vi "Event Handler.vi"(8 "error in (no error)":errorcluster, 10 "Stop Event Handler":refnum<user-event>, 11 "SwipeMenu in":refnum<class "SwipeMenu.lvclass">) -> (0 "error out":errorcluster)   [LabVIEW 2020, in "SwipeMenu.lvclass"]
doc: "The <b>Event Handler VI</b> is a dynamic dispatch VI that should be overwritten if events are needed to create the enhanced QControl. \n\nBy inheriting from the main Control.lvclass the overwritten <b>Event Handler VI</b> will be launched asynchronously in the initialization of the QControl.\n<b> </b> <b> </b>\n©2016 Q Software Innovations, LLC (QSI)\nwritten by Quentin Alldredge\nproduced in LabVIEW 2015\n\nsupport@qsoftwareinnovations.com\nwww.qsoftwareinnovations.com\n\nAll rights reserved.\n\nRedistribution and use in source and binary forms, with or without modification, are permitted provided that the following conditions are met:\n\n * Redistributions of source code must retain the above copyright notice, this list of conditions and the following disclaimer.\n * Redistributions in binary form must reproduce the above copyright notice, this list of conditions and the following disclaimer in the documentation and/or other materials provided with the distribution.\n * Neither the name of Q Software Innovations, LLC. nor the names of its contributors may be used to endorse or promote products derived from this software without specific prior written permission.\n\nTHIS SOFTWARE IS PROVIDED BY THE COPYRIGHT HOLDERS AND CONTRIBUTORS \"AS IS\" AND ANY EXPRESS OR IMPLIED WARRANTIES, INCLUDING, BUT NOT LIMITED TO, THE IMPLIED WARRANTIES OF MERCHANTABILITY AND FITNESS FOR A PARTICULAR PURPOSE ARE DISCLAIMED. IN NO EVENT SHALL THE COPYRIGHT OWNER OR CONTRIBUTORS BE LIABLE FOR ANY DIRECT, INDIRECT, INCIDENTAL, SPECIAL, EXEMPLARY, OR CONSEQUENTIAL DAMAGES (INCLUDING, BUT NOT LIMITED TO, PROCUREMENT OF SUBSTITUTE GOODS OR SERVICES; LOSS OF USE, DATA, OR PROFITS; OR BUSINESS INTERRUPTION) HOWEVER CAUSED AND ON ANY THEORY OF LIABILITY, WHETHER IN CONTRACT, STRICT LIABILITY, OR TORT (INCLUDING NEGLIGENCE OR OTHERWISE) ARISING IN ANY WAY OUT OF THE USE OF THIS SOFTWARE, EVEN IF ADVISED OF THE POSSIBILITY OF SUCH DAMAGE."
uses:
  SwipeMenu.lvclass
  Menu Cluster.ctl
  Demo Buttons/Test Button.ctl
  Demo Buttons/About Button.ctl
  Demo Buttons/Dismiss Popup.ctl
  Demo Buttons/QSI Button.ctl
  Demo Buttons/Checkbox Demo Button.ctl
  Demo Buttons/Dialogs Demo Button.ctl
  Demo Buttons/Example SubMenu Button.ctl
  Demo Buttons/Filter Clicks.ctl
  Demo Buttons/Listbox Demo Button.ctl
  Demo Buttons/OSK Demo Button.ctl
  Demo Buttons/Scrollbar Demo Button.ctl
  Demo Buttons/String Scrollbar Demo Button.ctl
  Demo Buttons/Swipe Scroll Button.ctl
  Demo Buttons/Swipe Select Button.ctl
  Left.ctl
  Right.ctl
  <vilib>/Utility/miscctls.llb/LVPointTypeDef.ctl
  SwipeMenu.lvclass/SwipeMenu.ctl
panel:
  in  "Left":T1
  in  "Menu Cluster":T2
  in  "Right":T17
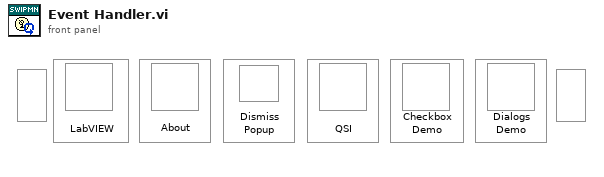
[diagram p1: front panel]
types:
  T1 = typedef "SwipeMenu.lvclass/Left.ctl" = bool
  T2 = typedef "SwipeMenu.lvclass/Menu Cluster.ctl" = cluster{"LabVIEW":T3, "About":T4, "Dismiss Popup":T5, "QSI":T6, "Checkboxes Demo":T7, "Dialog Demo":T8, "Submenu Demo":T9, "Filter Clicks":T10, "Listboxes Demo":T11, "OSK Demo":T12, "Scrollbar Demo":T13, "String Demo":T14, "Swipe Scroll":T15, "Swipe Select":T16, "LabVIEW 2":T3, "About 2":T4, "Dismiss Popup 2":T5, "QSI 2":T6, "Checkboxes Demo 2":T7, "Dialog Demo 2":T8, "Submenu Demo 2":T9, "Filter Clicks 2":T10, "Listboxes Demo 2":T11, "OSK Demo 2":T12, "Scrollbar Demo 2":T13, "String Demo 2":T14, "Swipe Scroll 2":T15, "Swipe Select 2":T16}
  T3 = typedef "Test Button.ctl" = bool
  T4 = typedef "About Button.ctl" = bool
  T5 = typedef "Dismiss Popup.ctl" = bool
  T6 = typedef "QSI Button.ctl" = bool
  T7 = typedef "Checkbox Demo Button.ctl" = bool
  T8 = typedef "Dialogs Demo Button.ctl" = bool
  T9 = typedef "Example SubMenu Button.ctl" = bool
  T10 = typedef "Filter Clicks.ctl" = bool
  T11 = typedef "Listbox Demo Button.ctl" = bool
  T12 = typedef "OSK Demo Button.ctl" = bool
  T13 = typedef "Scrollbar Demo Button.ctl" = bool
  T14 = typedef "String Scrollbar Demo Button.ctl" = bool
  T15 = typedef "Swipe Scroll Button.ctl" = bool
  T16 = typedef "Swipe Select Button.ctl" = bool
  T17 = typedef "SwipeMenu.lvclass/Right.ctl" = bool
  T18 = typedef "LVPointTypeDef.ctl" = cluster{"Horizontal":i16, "Vertical":i16}
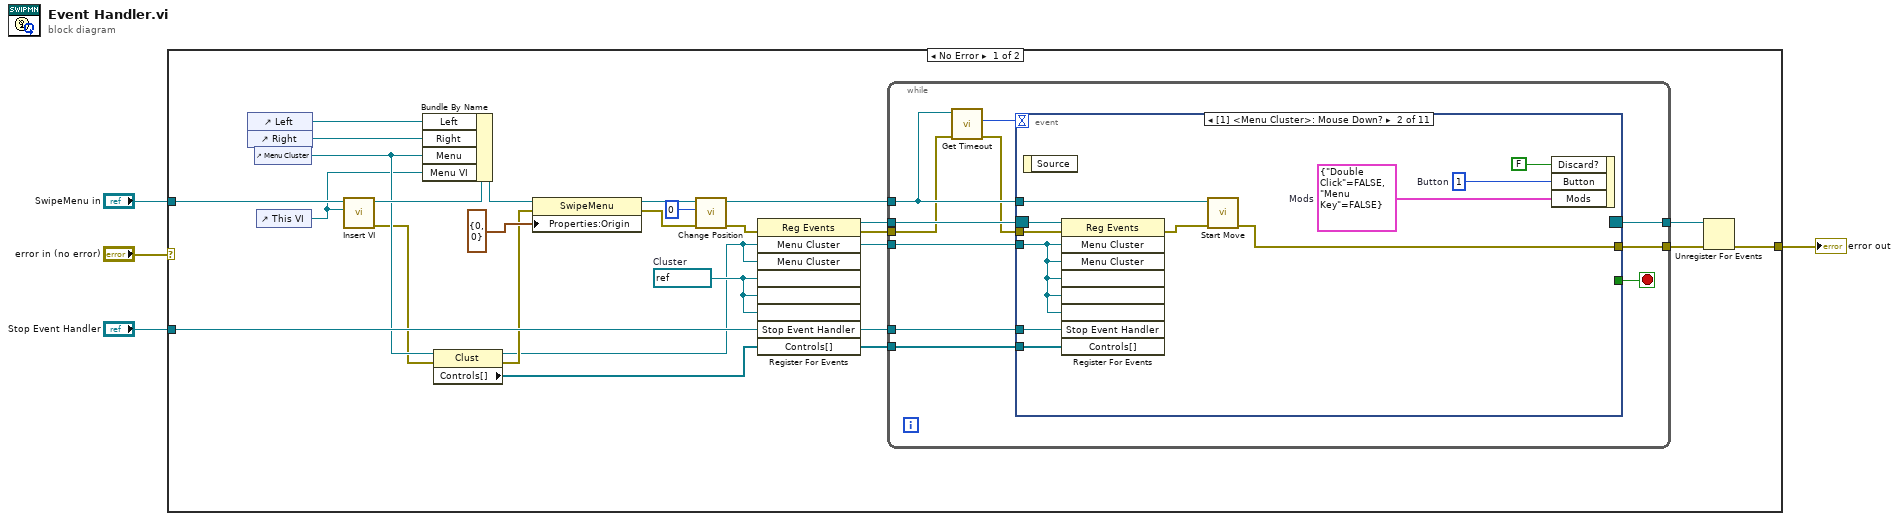
[diagram p0: block diagram]
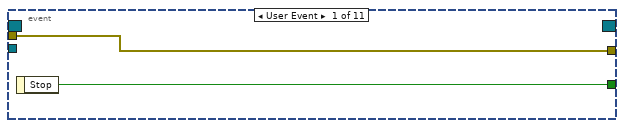
[diagram p2: hidden frame]
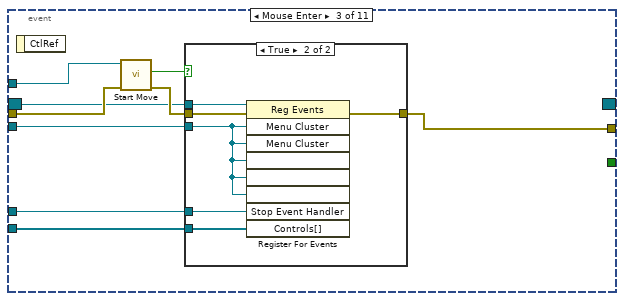
[diagram p3: hidden frame]
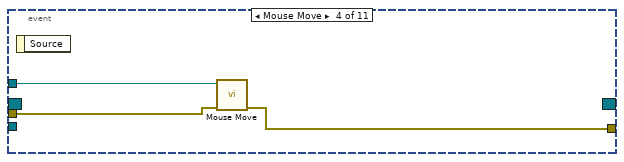
[diagram p5: hidden frame]
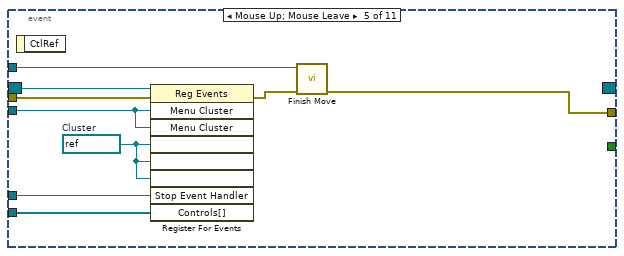
[diagram p6: hidden frame]
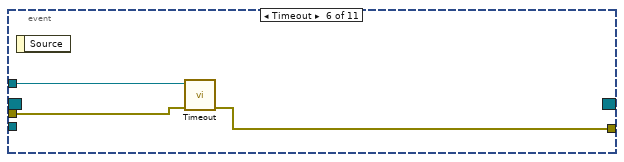
[diagram p7: hidden frame]
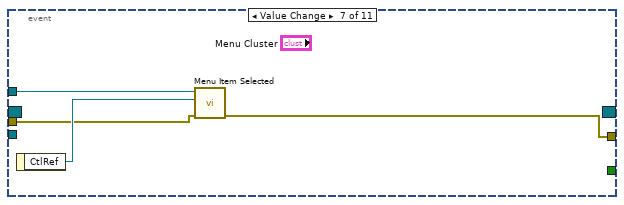
[diagram p8: hidden frame]
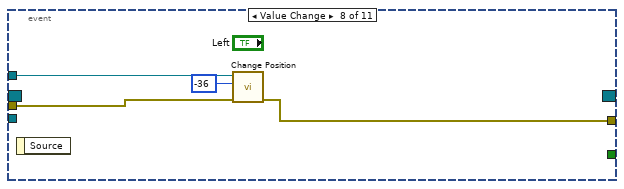
[diagram p9: hidden frame]
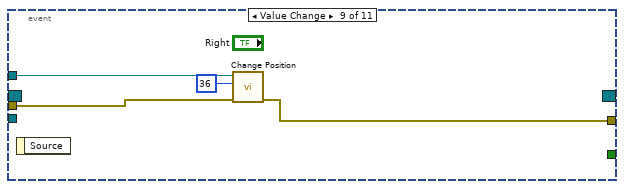
[diagram p10: hidden frame]
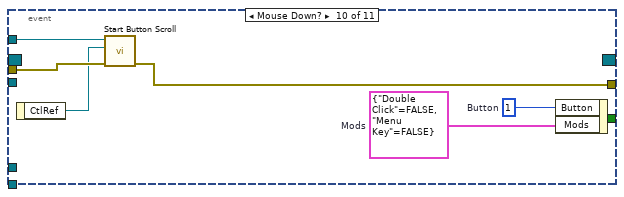
[diagram p11: hidden frame]
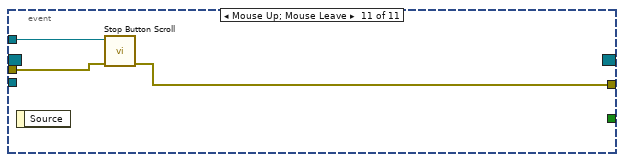
[diagram p12: hidden frame]
diagram:
  n1 = case shown="No Error" "error in (no error)" {
    selector: "error in (no error)" -> [_ w105]
    tunnel: [w25 w105] -> w3
    tunnel: "SwipeMenu in" -> [w20 _]
    tunnel: "Stop Event Handler" -> [w22 _]
    frame No Error {
      w23 = refnum<vi> refnum  # Cluster
      n2 = control-ref of="Left"() -> (w12:refnum<vi>)
      n3 = control-ref of="Right"() -> (w13:refnum<vi>)
      n4 = control-ref of="Menu Cluster"() -> (w17:refnum<vi>)
      n5 = control-ref of="This VI"() -> (w5:refnum<vi>)
      n6 = call-dynamic "Insert VI.vi"("VI Ref"=w5, "SubPanel in"=w20) -> ("error out"=w16:errorcluster, "SubPanel out"=w19:refnum<class "SwipeMenu.lvclass">)  [unwired: 8 in]
      n7 = Bundle By Name(cluster=w19, "Left"=w12, "Right"=w13, "Menu"=w17, "Menu VI"=w5) -> (w18:refnum<class "SwipeMenu.lvclass">)
      n8 = property class="Clust"(reference=w17, error in=w16) -> (reference out=w6:refnum<vi>, error out=w15:errorcluster, "Controls[]"=w14:refnum<vi>[])
      n9 = property class="SwipeMenu"(reference=w18, error in=w15, "Properties:Origin"=T18 {"Horizontal"=0, "Vertical"=0} ("Origin")) -> (reference out=w11:refnum<class "SwipeMenu.lvclass">, error out=w9:errorcluster)
      n10 = call "Change Position.vi"("error in (no error)"=w9, "Change Position"=i16 0, "SwipeMenu in"=w11) -> ("error out"=w8:errorcluster, "SwipeMenu out"=w10:refnum<class "SwipeMenu.lvclass">)  [unwired: 6 in, 1 out]
      n11 = register-events(error in=w8, w6, w6, w23, w23, w23, w22, w14) -> (reference out=w28:refnum<event-registration>, error out=w27:errorcluster)  [unwired: 1 in]
      n12 = while {
        tunnel: w28 -> [w39]
        tunnel: w27 -> [w30]
        tunnel: [w38] -> w26
        tunnel: [w36] -> w24
        tunnel: w10 -> [w32]
        tunnel: w22 -> [w35]
        tunnel: w6 -> [w34]
        tunnel: w14 -> [w29]
        stop <- w37 stop-if-true
        n13 = call "Get Timeout.vi"("error in (no error)"=w30, "SwipeMenu in"=w32) -> ("error out"=w31:errorcluster, "Timeout"=w33:i32)  [unwired: 7 in, 1 out]
        n14 = event shown="[1] <Menu Cluster>: Mouse Down?" {
          selector: w39 -> [_ w47 w55 _ w79 _ _ _ _ _ _]
          dyn-events: [_ _ _ _ _ _ _ _ _ _ _] -> w36
          timeout: w33 -> [_ _ _ _ _ _ _ _ _ _ _]
          tunnel: w32 -> [_ w52 w59 w71 w80 w83 w87 w91 w95 w101 w104]
          tunnel: w31 -> [w41 w51 w58 w70 w78 w82 w85 w90 w94 w100 w103]
          tunnel: [w41 w49 w53 w69 w74 w81 w84 w89 w93 w98 w102] -> w38
          tunnel: [w40 _ _ _ _ _ _ _ _ _ _] -> w37
          tunnel: w35 -> [_ w45 w61 _ w75 _ _ _ _ _ _]
          tunnel: w34 -> [_ w46 w60 _ w76 _ _ _ _ _ _]
          tunnel: w29 -> [_ w44 w54 _ w73 _ _ _ _ _ _]
          event User Event {
            n15 = event-data() -> ("Stop"=w40:bool)  [unwired: 1 in]
          }
          event Mouse Down? {
            w42 = cluster{"Double Click":bool, "Menu Key":bool} {"Double Click"=FALSE, "Menu Key"=FALSE}  # Mods
            w43 = u16 1  # Button
            n16 = event-data() -> ()  [unwired: 1 in, 1 out]
            n17 = register-events(reference=w47, error in=w51, w46, w46, w46, w46, w46, w45, w44) -> (error out=w50:errorcluster)  [unwired: 1 out]
            n18 = call "Start Move.vi"("error in (no error)"=w50, "SwipeMenu in"=w52) -> ("error out"=w49:errorcluster)  [unwired: 7 in, 2 out]
            n19 = event-data("Discard?"=FALSE, "Button"=w43, "Mods"=w42) -> ()  [unwired: 1 in, 1 out]
          }
          event Mouse Enter {
            n20 = event-data() -> ()  [unwired: 1 in, 1 out]
            n21 = call "Start Move.vi"("error in (no error)"=w58, "SwipeMenu in"=w59) -> ("error out"=w57:errorcluster, "Mouse Down?"=w56:bool)  [unwired: 7 in, 1 out]
            n22 = case shown="True" w56 {
              tunnel: w61 -> [_ w66]
              tunnel: w60 -> [_ w63]
              tunnel: w57 -> [w62 w68]
              tunnel: w55 -> [_ w67]
              tunnel: w54 -> [_ w65]
              tunnel: [w62 w64] -> w53
              frame False {
              }
              frame True {
                n23 = register-events(reference=w67, error in=w68, w63, w63, w63, w63, w63, w66, w65) -> (error out=w64:errorcluster)  [unwired: 1 out]
              }
            }
          }
          event Mouse Move {
            n24 = event-data() -> ()  [unwired: 1 in, 1 out]
            n25 = call "Mouse Move.vi"("error in (no error)"=w70, "SwipeMenu in"=w71) -> ("error out"=w69:errorcluster)  [unwired: 8 in, 1 out]
          }
          event Mouse Up; Mouse Leave {
            w72 = refnum<vi> refnum  # Cluster
            n26 = event-data() -> ()  [unwired: 1 in, 1 out]
            n27 = register-events(reference=w79, error in=w78, w76, w76, w72, w72, w72, w75, w73) -> (error out=w77:errorcluster)  [unwired: 1 out]
            n28 = call "Finish Move.vi"("error in (no error)"=w77, "SwipeMenu in"=w80) -> ("error out"=w74:errorcluster)  [unwired: 8 in, 1 out]
          }
          event Timeout {
            n29 = event-data() -> ()  [unwired: 1 in, 1 out]
            n30 = call "Timeout.vi"("error in (no error)"=w82, "SwipeMenu in"=w83) -> ("error out"=w81:errorcluster)  [unwired: 8 in, 1 out]
          }
          event Value Change {
            n31 = event-data() -> ("CtlRef"=w86:refnum<vi>)  [unwired: 1 in]
            n32 = call "Menu Item Selected.vi"("error in (no error)"=w85, "CtlRef"=w86, "SwipeMenu in"=w87) -> ("error out"=w84:errorcluster)  [unwired: 8 in]
          }
          event Value Change {
            n33 = event-data() -> ()  [unwired: 1 in, 1 out]
            n34 = call "Change Position.vi"("error in (no error)"=w90, "Change Position"=i16 -36, "SwipeMenu in"=w91) -> ("error out"=w89:errorcluster)  [unwired: 6 in, 2 out]
          }
          event Value Change {
            n35 = event-data() -> ()  [unwired: 1 in, 1 out]
            n36 = call "Change Position.vi"("error in (no error)"=w94, "Change Position"=i16 36, "SwipeMenu in"=w95) -> ("error out"=w93:errorcluster)  [unwired: 6 in, 2 out]
          }
          event Mouse Down? {
            w96 = cluster{"Double Click":bool, "Menu Key":bool} {"Double Click"=FALSE, "Menu Key"=FALSE}  # Mods
            w97 = u16 1  # Button
            n37 = event-data() -> ("CtlRef"=w99:refnum<vi>)  [unwired: 1 in]
            n38 = call "Start Button Scroll.vi"("error in (no error)"=w100, "CtlRef"=w99, "SwipeMenu in"=w101) -> ("error out"=w98:errorcluster)  [unwired: 7 in, 1 out]
            n39 = event-data("Button"=w97, "Mods"=w96) -> ()  [unwired: 1 in, 1 out]
          }
          event Mouse Up; Mouse Leave {
            n40 = event-data() -> ()  [unwired: 1 in, 1 out]
            n41 = call "Stop Button Scroll.vi"("error in (no error)"=w103, "SwipeMenu in"=w104) -> ("error out"=w102:errorcluster)  [unwired: 8 in, 1 out]
          }
        }
      }
      n42 = Unregister For Events(event registration refnum=w24, error in=w26) -> (error out=w25:errorcluster)
    }
    frame Error {
    }
  }
  "error out" <- w3
